vi "ReplaceList.vi"(10 "Old List":dbl[][](array[numeric]), 11 "New List":dbl[][](array[numeric])) -> (1 "Y":u32[](array[numeric]), 2 "X":u32[](array[numeric]))   [LabVIEW 2017, in "AODControl.lvlib"]
uses:
  AODControl.lvlib
  CodifyFrequency(Array).vi
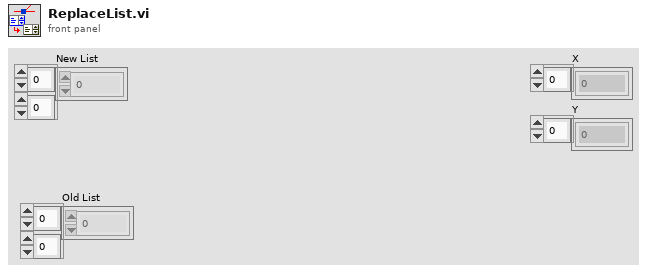
[diagram p1: front panel]
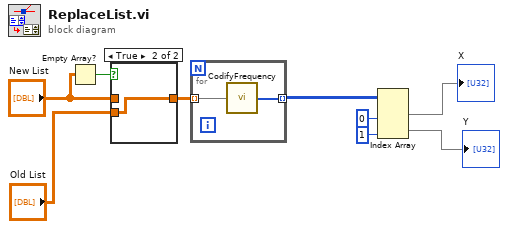
[diagram p0: block diagram]
diagram:
  n1 = Empty Array?(array="New List") -> (empty?=w4:bool)
  n2 = case shown="True" w4 {
    tunnel: [w10 w11] -> w2
    tunnel: "New List" -> [w10 _]
    tunnel: "Old List" -> [_ w11]
    frame False {
    }
    frame True {
    }
  }
  n3 = for {
    tunnel: w2 -> [w13] mode=indexing
    tunnel: [w12] -> w7 mode=indexing
    n4 = call-poly "CodifyFrequency.vi"("Array"=w13) -> ("Array 2"=w12:u32[])
  }
  n5 = Index Array(array=w7, index (col) #1=0 ("disabled index (col)"), index (col) #2=1 ("index (col)")) -> (element #1=→"X":u32[], element #2=→"Y":u32[])  [unwired: 2 in]
